vi "ConfigDataWidth 5034B.vi"(8 "error in (no error)":errorcluster, 11 "VISA resource name":refnum<visa-resource-name>) -> (0 "error out":errorcluster, 2 "Width":i32, 3 "VISA res name out":refnum<visa-resource-name>)   [LabVIEW 2012]
doc: "Configures the data width of the oscilloscope."
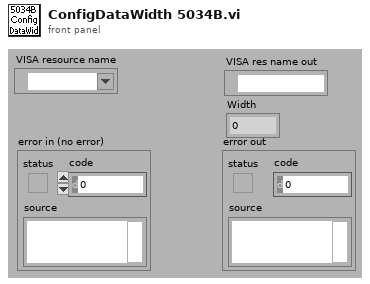
[diagram p1: front panel]
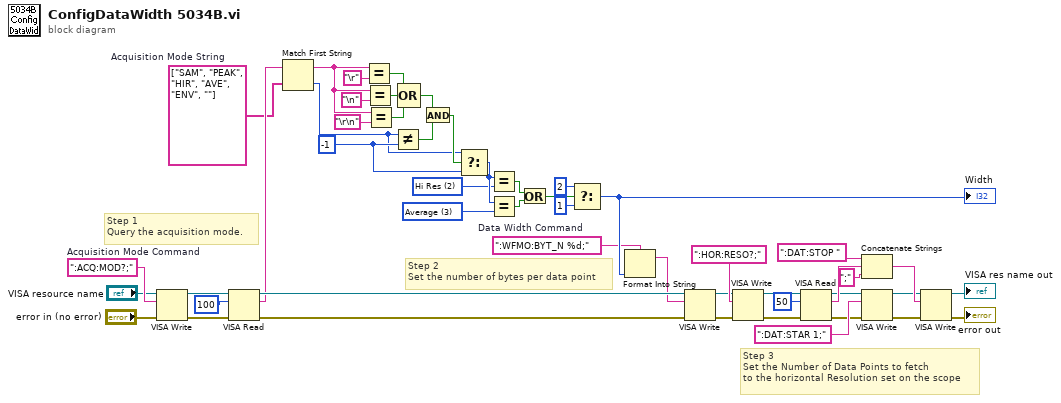
[diagram p0: block diagram]
diagram:
  w20 = u16 3 items=["Sample", "Peak Detect", "Hi Res", "Average", "Envelope"] ("Acquisition Mode (0:Sample)")
  w21 = u16 2 items=["Sample", "Peak Detect", "Hi Res", "Average", "WfmDB", "Envelope"] ("Acquisition Mode (0:Sample)")
  w44 = -1 ("y")
  w30 = ":WFMO:BYT_N %d;"  # Data Width Command
  w32 = string[] ["SAM", "PEAK", "HIR", "AVE", "ENV", ""]  # Acquisition Mode String
  w22 = ":ACQ:MOD?;"  # Acquisition Mode Command
  # "Step 3       \nSet the Number of Data Points to fetch\nto the horizontal Resolution set on the scope"
  # "Step 2       \nSet the number of bytes per data point"
  # "Step 1       \nQuery the acquisition mode."
  n1 = VISA Write(VISA resource name="VISA resource name", write buffer=w22, error in (no error)="error in (no error)") -> (VISA resource name out=w23:refnum<visa-resource-name>, error out=w24:errorcluster)  [unwired: 1 out]
  n2 = VISA Read(VISA resource name=w23, byte count=u32 100, error in (no error)=w24) -> (VISA resource name out=w49:refnum<visa-resource-name>, read buffer=w33:string, error out=w50:errorcluster)  [unwired: 1 out]
  n3 = Match First String(2:w32, 3:w33) -> (0:w43:i32, 1:w37:string)
  n4 = Equal?(x=w37, y="\r" ("Carriage Return Constant")) -> (x = y?=w38:bool)
  n5 = Equal?(x=w37, y="\n" ("Line Feed Constant")) -> (x = y?=w39:bool)
  n6 = Equal?(x=w37, y="\r\n" ("End of Line Constant")) -> (x = y?=w40:bool)
  n7 = Not Equal?(x=w43, y=w44) -> (x != y?=w42:bool)
  n8 = Compound Arithmetic op=OR(w38, w39, w40) -> (w41:bool)
  n9 = And(x=w41, y=w42) -> (x .and. y?=w45:bool)
  n10 = Select(t=w43, s=w45, f=w44) -> (s? t:f=w46:i32)
  n11 = Equal?(x=w46, y=w21) -> (x = y?=w26:bool)
  n12 = Equal?(x=w46, y=w20) -> (x = y?=w27:bool)
  n13 = Or(x=w26, y=w27) -> (x .or. y?=w47:bool)
  n14 = Select(t=2 ("f"), s=w47, f=1) -> (s? t:f=w31:i32)
  "Width" <- w31
  n15 = Format Into String(format string=w30, w31) -> (resulting string=w19:string)  [unwired: 2 in, 1 out]
  n16 = VISA Write(VISA resource name=w49, write buffer=w19, error in (no error)=w50) -> (VISA resource name out=w1:refnum<visa-resource-name>, error out=w5:errorcluster)  [unwired: 1 out]
  n17 = VISA Write(VISA resource name=w1, write buffer=":HOR:RESO?;", error in (no error)=w5) -> (VISA resource name out=w10:refnum<visa-resource-name>, error out=w9:errorcluster)  [unwired: 1 out]
  n18 = VISA Read(VISA resource name=w10, byte count=u32 50, error in (no error)=w9) -> (VISA resource name out=w11:refnum<visa-resource-name>, read buffer=w14:string, error out=w8:errorcluster)  [unwired: 1 out]
  n19 = Concatenate Strings(":DAT:STOP ", w14, ";") -> (w13:string)
  n20 = VISA Write(VISA resource name=w11, write buffer=":DAT:STAR 1;", error in (no error)=w8) -> (VISA resource name out=w12:refnum<visa-resource-name>, error out=w7:errorcluster)  [unwired: 1 out]
  n21 = VISA Write(VISA resource name=w12, write buffer=w13, error in (no error)=w7) -> (VISA resource name out=→"VISA res name out":refnum<visa-resource-name>, error out=→"error out":errorcluster)  [unwired: 1 out]
